vi "Path.vi"(8 "error in (no error)":errorcluster, 11 "Log in":refnum<class "Log.lvclass">) -> (0 "error out":errorcluster, 2 "Path":path, 3 "Log out":refnum<class "Log.lvclass">)   [LabVIEW 2026, in "TALOS.lvlib" / "Classes.lvlib" / "Log.lvclass"]
doc: "This VI returns the path to the log file."
uses:
  Log.lvclass
  Log.lvclass/Log.ctl
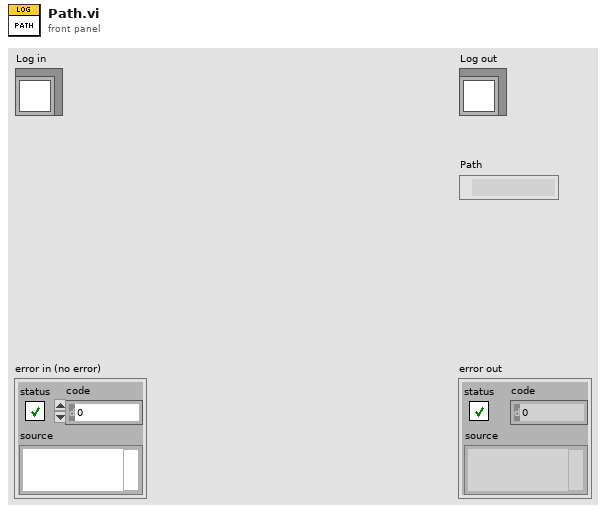
[diagram p1: front panel]
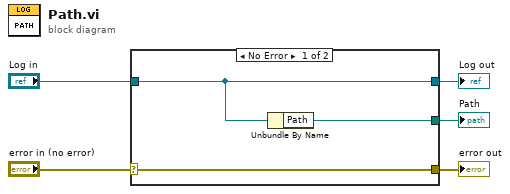
[diagram p0: block diagram]
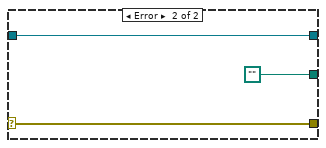
[diagram p2: hidden frame]
diagram:
  n1 = case shown="No Error" "error in (no error)" {
    selector: "error in (no error)" -> [w8 w11]
    tunnel: [w8 w11] -> w4
    tunnel: [w7 w10] -> w2
    tunnel: "Log in" -> [w7 w10]
    tunnel: [w6 path ""] -> w1
    frame No Error {
      n2 = Unbundle By Name(w7) -> ("Path"=w6:path)
    }
    frame Error {
    }
  }
  "error out" <- w4
  "Log out" <- w2
  "Path" <- w1
